vi "SAC-Compute ASTFs.vi"(0 "State":T3, 2 "Progress":refnum<vi>, 5 "Window":T1, 9 "Desired Fs":dbl) -> (15 "error out":errorcluster)   [LabVIEW 2020]
uses:
  Typedefs/SAC-State.ctl
  HRTF VIs/Typedefs/HRTF-Window.ctl
  HRTF VIs/Typedefs/HRTF-Window Type.ctl
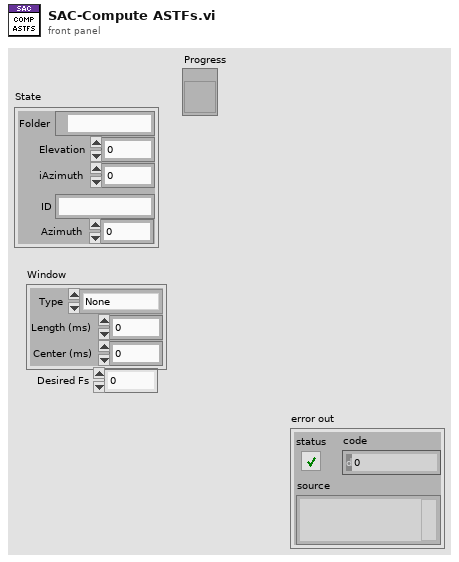
[diagram p1: front panel]
types:
  T1 = typedef "HRTF-Window.ctl" = cluster{"Type":T2, "Length (ms)":dbl, "Center (ms)":dbl}
  T2 = typedef "HRTF-Window Type.ctl" = enum16{"None", "Rectangle", "Hanning"}
  T3 = typedef "SAC-State.ctl" = cluster{"Folder":path, "Elevation":dbl, "iAzimuth":i32, "ID":string, "Azimuth":dbl}
  T4 = enum8{"Enabled", "Disabled", "Disabled and Grayed Out"}
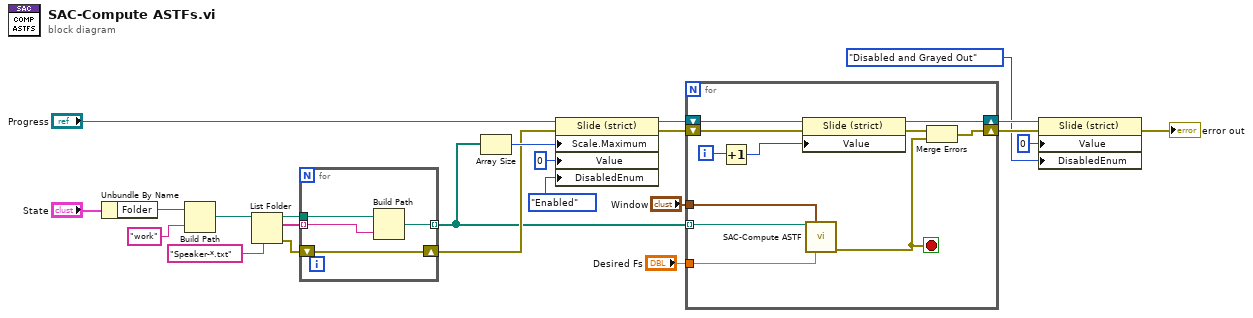
[diagram p0: block diagram]
diagram:
  n1 = Unbundle By Name("State") -> ("Folder"=w22:path)
  n2 = Build Path(base path=w22, name or relative path="work") -> (appended path=w20:path)
  n3 = List Folder(path=w20, pattern="Speaker-*.txt") -> (path out=w18:path, filenames=w17:string[], error out=w16:errorcluster)  [unwired: 2 in, 1 out]
  n4 = for {
    tunnel: w18 -> [w27]
    tunnel: w17 -> [w26] mode=indexing
    tunnel: [w25] -> w11 mode=indexing
    shift-right: [w24] -> w12
    shift-left: w16 -> [w24]
    n5 = Build Path(base path=w27, name or relative path=w26) -> (appended path=w25:path)
  }
  n6 = Array Size(array=w11) -> (size(s)=w14:i32)
  n7 = property class="Slide (strict)"(reference="Progress", error in=w12, "Scale.Maximum"=w14, "Value"=u8 0, "DisabledEnum"=T4."Enabled" ("Disabled")) -> (reference out=w10:refnum<vi>, error out=w9:errorcluster)
  n8 = for {
    tunnel: w11 -> [w28] mode=indexing
    shift-right: [w37] -> w7
    shift-left: w10 -> [w38]
    shift-right: [w29] -> w6
    shift-left: w9 -> [w36]
    tunnel: "Window" -> [w33]
    tunnel: "Desired Fs" -> [w32]
    i -> [w35]
    stop <- w30 stop-if-true
    n9 = Increment(x=w35) -> (x+1=w34:i32)
    n10 = property class="Slide (strict)"(reference=w38, error in=w36, "Value"=w34) -> (reference out=w37:refnum<vi>, error out=w31:errorcluster)
    n11 = call "SAC-Compute ASTF.vi"("speaker path"=w28, "Window"=w33, "Desired Fs"=w32) -> ("error out"=w30:errorcluster)  [unwired: 12 in]
    n12 = Merge Errors(w31, w30) -> (w29:errorcluster)
  }
  n13 = property class="Slide (strict)"(reference=w7, error in=w6, "Value"=u8 0, "DisabledEnum"=T4."Disabled and Grayed Out" ("Disabled")) -> (error out=→"error out":errorcluster)  [unwired: 1 out]
